vi "Set Trigger Mode.vi"(8 "error in (no error)":errorcluster, 10 "Trigger Mode":enum16{"Input Mode", "Output Mode"}(ring), 11 "FW102C in":i32) -> (0 "error out":errorcluster, 3 "FW102C out":i32)   [LabVIEW 2017, in "Colour Wheel.lvlib" / "Thorlabs_FW102C.lvlib"]
doc: "trig=0 Sets the external trigger to the input mode, Respond to an active low pulse by advancing position by 1\ntrig=1 Sets the external trigger to the output mode, Generate an active high pulse when selected position arrived at"
uses:
  Thorlabs_FW102C.lvlib
  Library/FilterWheel102_win32.dll
  Library/FilterWheel102_win64.dll
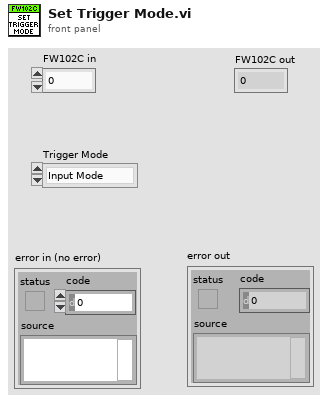
[diagram p1: front panel]
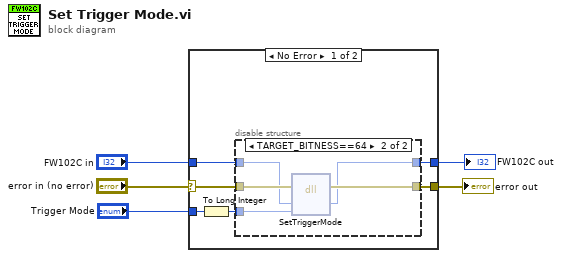
[diagram p0: block diagram]
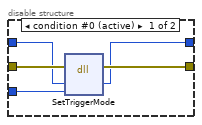
[diagram p2: hidden frame]
diagram:
  n1 = case shown="No Error" "error in (no error)" {
    selector: "error in (no error)" -> [w11 w22]
    tunnel: [w10 w22] -> w5
    tunnel: "FW102C in" -> [w9 w23]
    tunnel: [w8 w23] -> w2
    tunnel: "Trigger Mode" -> [w7 _]
    frame No Error {
      n2 = To Long Integer(number=w7) -> (32bit integer=w6:i32)
      n3 = disable-structure shown="TARGET_BITNESS==64" {
        disable-tunnel: w11 -> [w16 w21]
        disable-tunnel: [w15 w20] -> w10
        disable-tunnel: w9 -> [w14 w19]
        disable-tunnel: [w13 w18] -> w8
        disable-tunnel: w6 -> [w12 w17]
        frame condition #0 (active) {
          n4 = dll-call lib="C:/Project Work/icl-optical-software-rewrite/Optical Software Code Simplified/Modules/Colour Wheel/Thorlabs_FW102C/Library/FilterWheel102_win32.dll" fn="SetTriggerMode"(error in=w16, "hdl"=w14, "trigger mode"=w12) -> (error out=w15:errorcluster, "hdl"=w13:i32)  [unwired: 4 in, 1 out]
        }
        frame condition #1 {
          n5 = dll-call lib="C:/Project Work/icl-optical-software-rewrite/Optical Software Code Simplified/Modules/Colour Wheel/Thorlabs_FW102C/Library/FilterWheel102_win64.dll" fn="SetTriggerMode"(error in=w21, "hdl"=w19, "trigger mode"=w17) -> (error out=w20:errorcluster, "hdl"=w18:i32)  [unwired: 4 in, 1 out]
        }
      }
    }
    frame Error {
    }
  }
  "error out" <- w5
  "FW102C out" <- w2
